vi "4155C Take Sample.vi"(7 "Emergency Stop":refnum<vi>, 8 "error in (no error)":errorcluster, 9 "Vd":dbl min=-100.0 max=100.0 format="%.2f", 10 "Vg":dbl min=-100.0 max=100.0 format="%.2f", 11 "VISA resource name in":refnum<visa-resource-name>) -> (0 "error out":errorcluster, 1 "Id":dbl[](array[numeric]) format="%.2f", 2 "Ig":dbl[](array[numeric]) format="%.2f", 3 "VISA Resource Name out":refnum<visa-resource-name>, 4 "Is":dbl[](array[numeric]) format="%.2f", 5 "Time":dbl[](array[numeric]) format="%.2f")   [LabVIEW 2016]
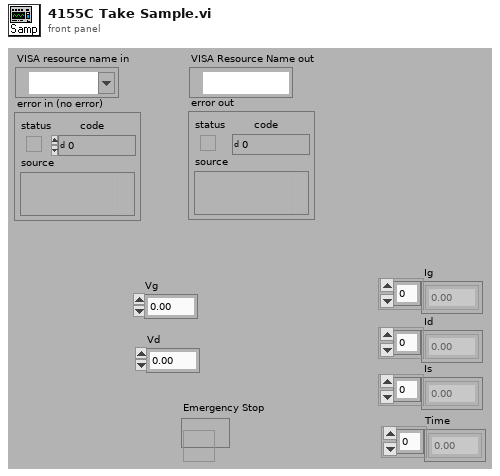
[diagram p1: front panel]
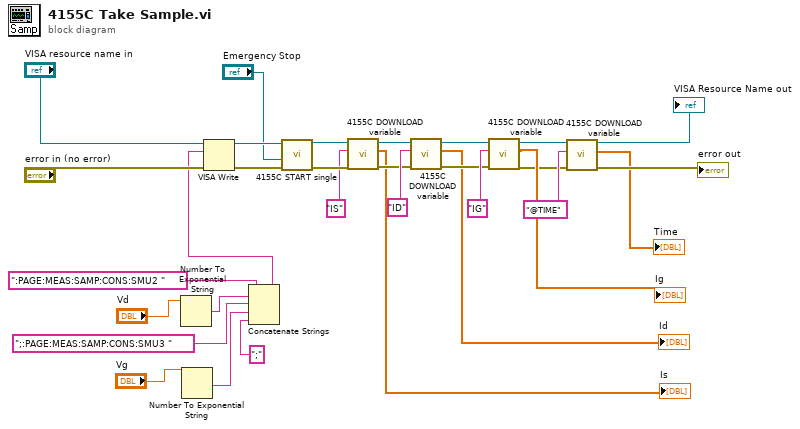
[diagram p0: block diagram]
diagram:
  n1 = Number To Exponential String(number="Vd") -> (E-format string=w30:string)  [unwired: 3 in]
  n2 = Number To Exponential String(number="Vg") -> (E-format string=w27:string)  [unwired: 3 in]
  n3 = Concatenate Strings(":PAGE:MEAS:SAMP:CONS:SMU2 " ("write buffer (\"\")"), w30, ";:PAGE:MEAS:SAMP:CONS:SMU3 " ("write buffer (\"\")"), w27, ";" ("Substring")) -> (w24:string)
  n4 = VISA Write(VISA resource name="VISA resource name in", write buffer=w24, error in (no error)="error in (no error)") -> (VISA resource name out=w22:refnum<visa-resource-name>, error out=w21:errorcluster)  [unwired: 1 out]
  n5 = call "4155C START single.vi"("error in (no error)"=w21, "Emergency Stop"="Emergency Stop", "VISA resource name in"=w22) -> ("error out"=w18:errorcluster, "VISA Resource Name out"=w19:refnum<visa-resource-name>)  [unwired: 3 in]
  n6 = call "4155C DOWNLOAD variable.vi"("error in (no error)"=w18, "Variable name"="IS", "VISA resource name in"=w19) -> ("error out"=w15:errorcluster, "Output data"=→"Is":dbl[], "VISA Resource Name out"=w14:refnum<visa-resource-name>)  [unwired: 2 in]
  n7 = call "4155C DOWNLOAD variable.vi"("error in (no error)"=w15, "Variable name"="ID", "VISA resource name in"=w14) -> ("error out"=w12:errorcluster, "Output data"=→"Id":dbl[], "VISA Resource Name out"=w11:refnum<visa-resource-name>)  [unwired: 2 in]
  n8 = call "4155C DOWNLOAD variable.vi"("error in (no error)"=w12, "Variable name"="IG", "VISA resource name in"=w11) -> ("error out"=w4:errorcluster, "Output data"=→"Ig":dbl[], "VISA Resource Name out"=w5:refnum<visa-resource-name>)  [unwired: 2 in]
  n9 = call "4155C DOWNLOAD variable.vi"("error in (no error)"=w4, "Variable name"="@TIME", "VISA resource name in"=w5) -> ("error out"=→"error out":errorcluster, "Output data"=→"Time":dbl[], "VISA Resource Name out"=→"VISA Resource Name out":refnum<visa-resource-name>)  [unwired: 2 in]
